vi "shooter.vi"(8 "axis 4":dbl, 9 "axis 3 (throttle)":dbl) -> ()   [LabVIEW 2012]
panel:
  out "Axis 3 (throttle) 2":dbl
  out "Axis 3 (throttle)":dbl
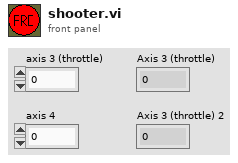
[diagram p1: front panel]
types:
  T1 = typedef "WPI_MotorControlDeviceRef.ctl" = cluster{"DeviceStatus":errorcluster, "Type":enum16{"PWM", "CAN"}, "PWM":cluster{"Digital Module":T2, "PWM Channel":T3, "DeadBand":T4}, "CAN":cluster{"Device Number":u8, "Control Mode":T5, "Semaphore":T6, "Max Vout":dbl}, "Invert":bool, "TransformRef":T7, "InvTransformRef":T7}
  T2 = typedef "FPGA_TypedefDigitalModule.ctl" = enum16{"Digital Module 1", "Digital Module 2"}
  T3 = typedef "FPGA_DIOPWMChannel.ctl" = enum8{"PWM 1", "PWM 2", "PWM 3", "PWM 4", "PWM 5", "PWM 6", "PWM 7", "PWM 8", "PWM 9", "PWM 10", "Invalid"}
  T4 = typedef "WPI_PWMDeadband.ctl" = cluster{"Name":string, "maxPositivePwm":i32, "minPositivePwm":i32, "centerPwm":i32, "maxNegativePwm":i32, "minNegativePwm":i32, "angularRange":u16}
  T5 = typedef "WPI_CANJaguar_ControlMode.ctl" = enum8{"Percent VBus", "Current", "Speed", "Position", "Voltage"}
  T6 = typedef "Semaphore RefNum" = refnum<k1>
  T7 = typedef "WPI_PWMTransform_ConPane.ctl" = refnum<vi>
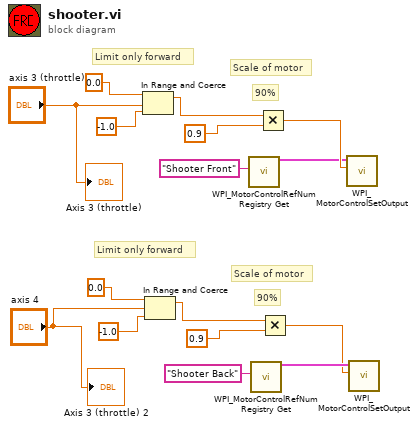
[diagram p0: block diagram]
diagram:
  # "Scale of motor"
  # "Scale of motor"
  # "Limit only forward"
  # "90%"
  # "Limit only forward"
  # "90%"
  n1 = In Range and Coerce(upper limit=0.0, x="axis 3 (throttle)", lower limit=-1.0) -> (coerced(x)=w7:dbl)  [unwired: 1 out]
  n2 = In Range and Coerce(upper limit=0.0, x="axis 4", lower limit=-1.0) -> (coerced(x)=w10:dbl)  [unwired: 1 out]
  n3 = call <vilib>:"WPI_MotorControlRefNum Registry Get.vi"("refnum name"="Shooter Front") -> ("MotorControlDevRef"=w1:T1)  [unwired: 9 in, 1 out]
  n4 = call <vilib>:"WPI_MotorControlRefNum Registry Get.vi"("refnum name"="Shooter Back") -> ("MotorControlDevRef"=w15:T1)  [unwired: 9 in, 1 out]
  n5 = Multiply(x=w7, y=0.9) -> (x*y=w3:dbl)
  n6 = Multiply(x=w10, y=0.9) -> (x*y=w13:dbl)
  n7 = call <vilib>:"WPI_MotorControlSetOutput.vi"("Output"=w3, "MotorControlDevRef"=w1) -> ()  [unwired: 7 in, 3 out]
  n8 = call <vilib>:"WPI_MotorControlSetOutput.vi"("Output"=w13, "MotorControlDevRef"=w15) -> ()  [unwired: 7 in, 3 out]
  "Axis 3 (throttle)" <- "axis 3 (throttle)"
  "Axis 3 (throttle) 2" <- "axis 4"
